vi "GE 5565PIORC.DMA.Block.In-Place Read (DBL).vi"(5 "byte order (big-endian)":T1(ring), 7 "count (-1: all)":i32=-1, 8 "error in (no error)":errorcluster, 9 "data in":dbl[](array[numeric]), 10 "Block Descriptor in":T2 {"descriptor params"."data ptr (lower)" format="%.0x"; "descriptor params"."data ptr (upper)" format="%.0x"; "descriptor params"."data size" format="%.0x"; "descriptor params"."next descriptor ptr" format="%.0x"; "descriptor size" format="%08x"; "descriptor ptr (RFM)" format="%08x"; "descriptor ptr (VISA)" format="%08x"}, 11 "GE 5565PIORC in":refnum<class "GE 5565PIORC.lvclass">) -> (0 "error out":errorcluster, 1 "data out":dbl[](array[numeric]), 2 "Block Descriptor out":T2 {"descriptor params"."data ptr (lower)" format="%.0x"; "descriptor params"."data ptr (upper)" format="%.0x"; "descriptor params"."data size" format="%.0x"; "descriptor params"."next descriptor ptr" format="%.0x"; "descriptor size" format="%08x"; "descriptor ptr (RFM)" format="%08x"; "descriptor ptr (VISA)" format="%08x"}, 3 "GE 5565PIORC out":refnum<class "GE 5565PIORC.lvclass">)   [LabVIEW 2024, in "GE 5565PIORC.lvclass"]
doc: "Reads <B>count</B> elements from the provided <B>Block Descriptor</B> into the provided <B>data</B> array. The number of elements transferred will be either <B>count</B> or the number of elements in <B>data</B>, whichever is smaller."
uses:
  GE 5565PIORC.lvclass
  Typedefs/GE 5565PIORC.Typedef.DMA Block Descriptor.ctl
  Typedefs/GE 5565PIORC.Typedef.DMA Block Descriptor Params.ctl
  <vilib>/Instr/_visa.llb/VISA Register Access Address Space.ctl
  GE 5565PIORC.lvclass/GE 5565PIORC.ctl
  GE 5565PIORC.VISA.Return Handler.vi
  <vilib>/Utility/error.llb/Error Cluster From Error Code.vi
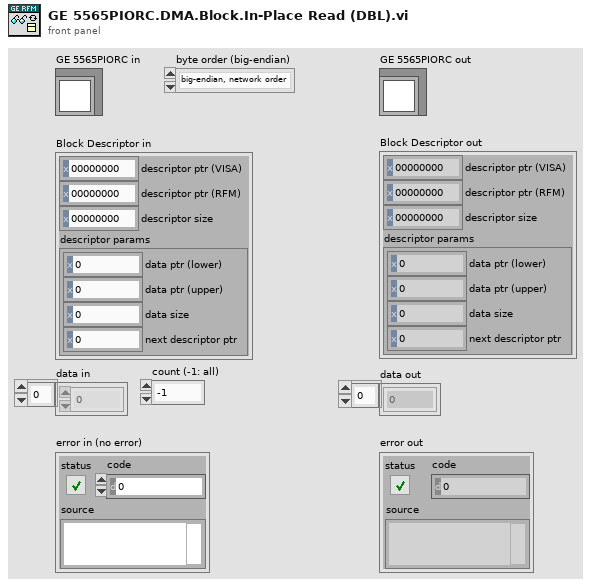
[diagram p1: front panel]
types:
  T1 = enum16{"big-endian, network order", "native, host order", "little-endian"}
  T2 = typedef "GE 5565PIORC.lvclass/GE 5565PIORC.Typedef.DMA Block Descriptor.ctl" = cluster{"descriptor ptr (VISA)":u32, "descriptor ptr (RFM)":u32, "descriptor size":u32, "descriptor params":T3}
  T3 = typedef "GE 5565PIORC.lvclass/GE 5565PIORC.Typedef.DMA Block Descriptor Params.ctl" = cluster{"data ptr (lower)":u32, "data ptr (upper)":u32, "data size":u32, "next descriptor ptr":u32}
  T4 = typedef "VISA Register Access Address Space.ctl" = u16
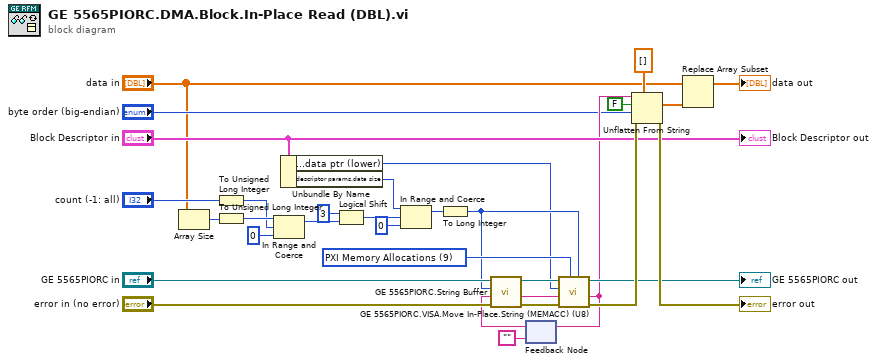
[diagram p0: block diagram]
diagram:
  w18 = T4 9 items=["VXI/VME A16"=1, "VXI/VME A24"=2, "VXI/VME A32"=3, "VXI/VME A64"=4, "PXI Memory Allocations"=9, "PXI Configuration"=10, "PXI BAR0"=11, "PXI BAR1"=12, "PXI BAR2"=13, "PXI BAR3"=14, "PXI BAR4"=15, "PXI BAR5"=16] ("address space")
  n1 = Array Size(array="data in") -> (size(s)=w28:i32)
  n2 = To Unsigned Long Integer(number="count (-1: all)") -> (unsigned 32bit integer=w10:u32)
  n3 = To Unsigned Long Integer(number=w28) -> (unsigned 32bit integer=w17:u32)
  n4 = In Range and Coerce(upper limit=w17, x=w10, lower limit=u32 0) -> (coerced(x)=w16:u32)  [unwired: 1 out]
  n5 = Unbundle By Name("Block Descriptor in") -> ("descriptor params.data ptr (lower)"=w2:u32, "descriptor params.data size"=w13:u32)
  n6 = Logical Shift(y=i16 3, x=w16) -> (x << y=w15:u32)
  n7 = In Range and Coerce(upper limit=w13, x=w15, lower limit=u32 0) -> (coerced(x)=w7:u32)  [unwired: 1 out]
  n8 = To Long Integer(number=w7) -> (32bit integer=w6:i32)
  n9 = feedback #1("" ("data out")) -> (w5:string)
  n10 = call "GE 5565PIORC.String Buffer.vi"("error in (no error)"="error in (no error)", "string buffer in"=w5, "minimum size"=w6, "GE 5565PIORC in"="GE 5565PIORC in") -> ("error out"=w24:errorcluster, "string buffer out"=w23:string, "GE 5565PIORC out"=w25:refnum<class "GE 5565PIORC.lvclass">)  [unwired: 5 in]
  n11 = call "GE 5565PIORC.VISA.Move In-Place.String (MEMACC) (U8).vi"("count (-1: all)"=w6, "address space"=w18, "error in (no error)"=w24, "data in"=w23, "offset"=w2, "GE 5565PIORC in"=w25) -> ("error out"=w32:errorcluster, "data out"=w4:string, "GE 5565PIORC out"=→"GE 5565PIORC out":refnum<class "GE 5565PIORC.lvclass">)  [unwired: 3 in]
  n12 = feedback-in #1(w4) -> ()
  n13 = Unflatten From String(type=dbl[] [], binary string=w4, data includes array or string size? (T)=FALSE, byte order (0:big-endian, network order)="byte order (big-endian)", error in (no error)=w32) -> (value=w22:dbl[], error out=→"error out":errorcluster)  [unwired: 1 out]
  n14 = Replace Array Subset(array="data in", new element=w22) -> (→"data out":dbl[])  [unwired: 1 in]
  "Block Descriptor out" <- "Block Descriptor in"
